vi "CIE-Apply Probe Tube Smoothing.vi"(0 "Vprb/Vdac":dbl[](array[numeric]), 5 "Frequency (Hz)":dbl[](array[numeric]), 7 "Probe Tube Path":path, 9 "Override?":bool, 11 "error in (no error)":errorcluster) -> (4 "Smoothed Mag":dbl[](array[numeric]), 8 "Smoothed?":bool, 10 "Smooth Params":T1={"Method"=enum."None", "MA"={"Iterations"=100, "Length"=3}, "Loess"={"Length"=21, "Type"=enum."Quadratic", "Robust"=TRUE}} {"Loess"."Length" min=1 step=1; "MA"."Length" min=1 step=1; "MA"."Iterations" min=1 step=1}, 15 "error out":errorcluster)   [LabVIEW 2020]
uses:
  Type Defs/Cal-Smoothing Parameters.ctl
  epl-vi-lib/Utility VIs/Comparison VIs/Approx Equal (1D).vi
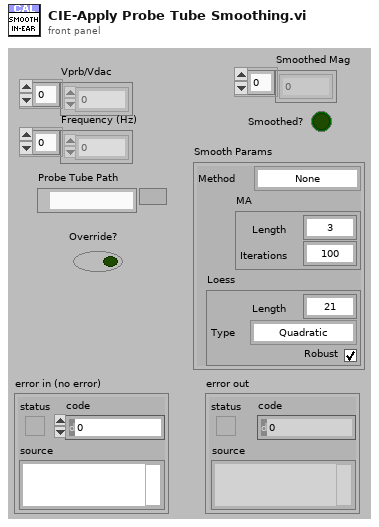
[diagram p1: front panel]
types:
  T1 = typedef "Cal-Smoothing Parameters.ctl" = cluster{"Method":enum16{"None", "Moving average", "Loess"}, "MA":cluster{"Iterations":i32, "Length":i32}, "Loess":cluster{"Length":i32, "Type":enum16{"Linear", "Quadratic"}, "Robust":bool}}
  T2 = cluster{"Length":i32, "Type":enum16{"Linear", "Quadratic"}, "Robust":bool}
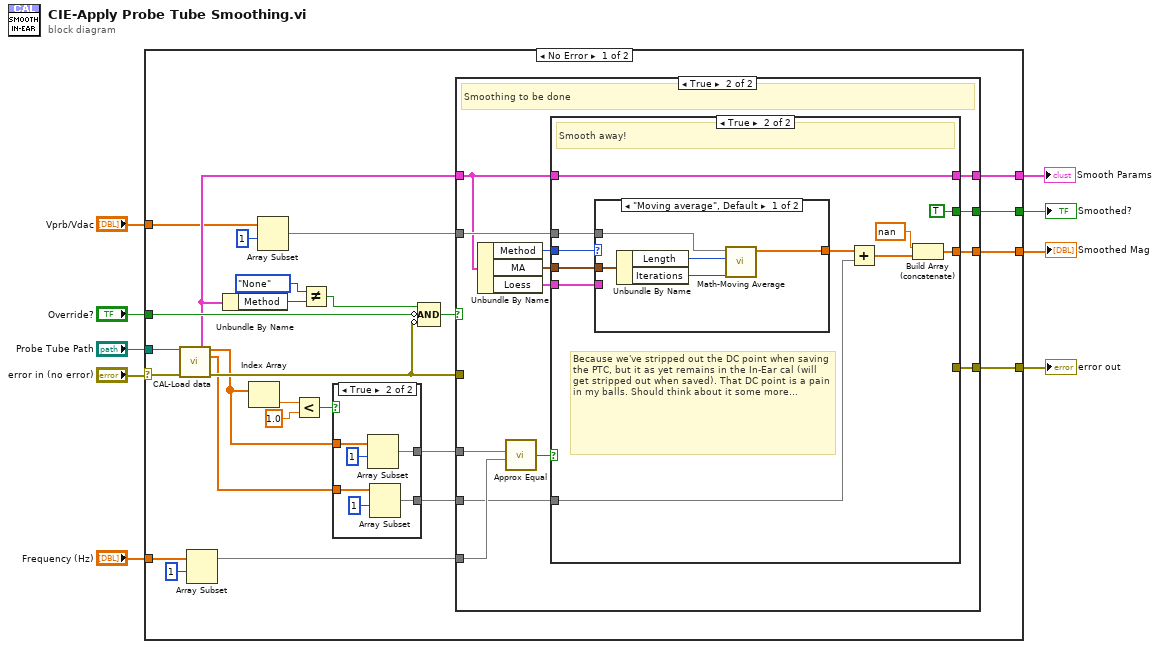
[diagram p0: block diagram]
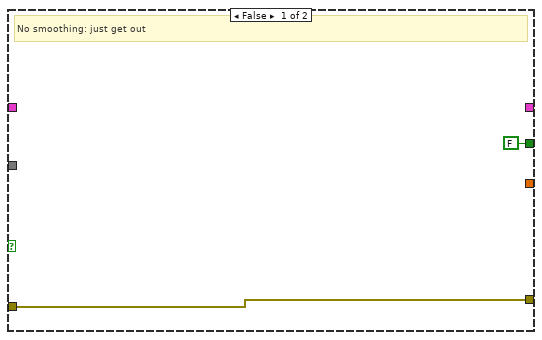
[diagram p3: hidden frame]
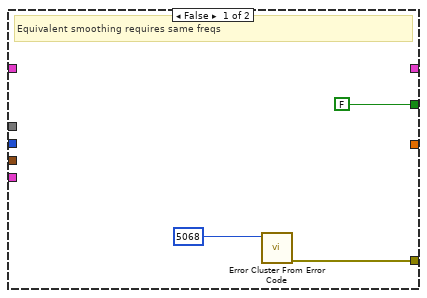
[diagram p4: hidden frame]
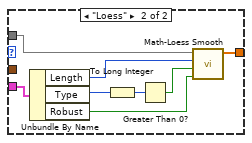
[diagram p5: hidden frame]
diagram:
  n1 = case shown="No Error" "error in (no error)" {
    selector: "error in (no error)" -> [w35 w86]
    tunnel: [w30 w86] -> w8
    tunnel: "Probe Tube Path" -> [w34 _]
    tunnel: "Override?" -> [w27 _]
    tunnel: [w29 _] -> w5
    tunnel: "Frequency (Hz)" -> [w28 _]
    tunnel: "Vprb/Vdac" -> [w18 _]
    tunnel: [w23 _] -> w2
    tunnel: [w22 _] -> w1
    frame No Error {
      n2 = call "CAL-Load data.vi"("user path"=w34, "error in (no error)"=w35) -> ("Smooth Params"=w24:T1, "Frequency (Hz)"=w13:dbl[], "Mag"=w12:dbl[], "error out"=w31:errorcluster)  [unwired: 6 in, 4 out]
      n3 = Array Subset(array=w28, index=1) -> (w21:dbl[])  [unwired: 1 in]
      n4 = Unbundle By Name(w24) -> ("Method"=w26:enum16{"None", "Moving average", "Loess"})
      n5 = Index Array(array=w13) -> (element=w16:dbl)  [unwired: 1 in]
      n6 = Array Subset(array=w18, index=1) -> (w17:dbl[])  [unwired: 1 in]
      n7 = Less?(x=w16, y=1.0) -> (x < y?=w14:bool)
      n8 = Not Equal?(x=enum16{"None", "Moving average", "Loess"}."None", y=w26) -> (x != y?=w25:bool)
      n9 = case shown="True" w14 {
        tunnel: w13 -> [w37 w42]
        tunnel: w12 -> [w36 w39]
        tunnel: [w37 w41] -> w11
        tunnel: [w36 w38] -> w10
        frame False {
        }
        frame True {
          n10 = Array Subset(array=w42, index=1) -> (w41:dbl[])  [unwired: 1 in]
          n11 = Array Subset(array=w39, index=1) -> (w38:dbl[])  [unwired: 1 in]
        }
      }
      n12 = Compound Arithmetic op=AND(w25, invert w27, invert w31) -> (w32:bool)
      n13 = case shown="True" w32 {
        tunnel: w10 -> [_ w56]
        tunnel: w31 -> [w45 _]
        tunnel: [w45 w54] -> w30
        tunnel: [FALSE w49] -> w29
        tunnel: w21 -> [_ w58]
        tunnel: w17 -> [_ w55]
        tunnel: w24 -> [_ w47]
        tunnel: [_ w50] -> w23
        tunnel: [_ w48] -> w22
        tunnel: w11 -> [_ w46]
        frame False {
          # "No smoothing: just get out"
        }
        frame True {
          # "Smoothing to be done"
          n14 = Unbundle By Name(w47) -> ("Method"=w53:enum16{"None", "Moving average", "Loess"}, "MA"=w52:cluster{"Iterations":i32, "Length":i32}, "Loess"=w51:T2)
          n15 = call-poly "Approx Equal.vi"("Y"=w58, "X"=w46) -> ("X approx Y?"=w57:bool)  [unwired: 4 in]
          n16 = case shown="True" w57 {
            tunnel: w56 -> [_ w64]
            tunnel: w55 -> [_ w69]
            tunnel: [w61 _] -> w54
            tunnel: w53 -> [_ w72]
            tunnel: w52 -> [_ w71]
            tunnel: w51 -> [_ w70]
            tunnel: [_ w63] -> w50
            tunnel: [FALSE TRUE] -> w49
            tunnel: [_ w65] -> w48
            tunnel: w47 -> [_ w65]
            frame False {
              # "Equivalent smoothing requires same freqs"
              n17 = call <vilib>:"Error Cluster From Error Code.vi"("error code (0)"=5068) -> ("error out"=w61:errorcluster)  [unwired: 8 in]
            }
            frame True {
              # "Because we've stripped out the DC point when saving the PTC, but it as yet remains in the In-Ear cal (will get stripped out when saved). That DC point is a pain in my balls. Should think about it some more..."
              # "Smooth away!"
              n18 = case shown="\"Moving average\", Default" w72 {
                tunnel: w71 -> [w75 _]
                tunnel: w70 -> [_ w80]
                tunnel: w69 -> [w74 w78]
                tunnel: [w73 w79] -> w68
                frame "Moving average", Default {
                  n19 = Unbundle By Name(w75) -> ("Length"=w76:i32, "Iterations"=w77:i32)
                  n20 = call "Math-Moving Average.vi"("Iterations"=w77, "Length"=w76, "Array in"=w74) -> ("Array out"=w73:dbl[])  [unwired: 8 in]
                }
                frame "Loess" {
                  n21 = Unbundle By Name(w80) -> ("Length"=w83:i32, "Type"=w81:enum16{"Linear", "Quadratic"}, "Robust"=w85:bool)
                  n22 = To Long Integer(number=w81) -> (32bit integer=w84:i32)
                  n23 = Greater Than 0?(x=w84) -> (x > 0?=w82:bool)
                  n24 = call "Math-Loess Smooth.vi"("Robust?"=w85, "Quadratic?"=w82, "Span"=w83, "Array"=w78) -> ("Smoothed Array"=w79:dbl[])  [unwired: 7 in]
                }
              }
              n25 = Add(x=w68, y=w64) -> (x+y=w66:dbl[])
              n26 = Build Array (concatenate)(nan, w66) -> (w63:dbl[])
            }
          }
        }
      }
    }
    frame Error {
    }
  }
  "error out" <- w8
  "Smoothed Mag" <- w2
  "Smoothed?" <- w5
  "Smooth Params" <- w1
